vi "DrawCircle.vi"(6 "Phase":dbl step=0.1, 8 "Eccentricity":dbl min=0.0 step=0.05, 9 "No Of Points":i32, 10 "Radius":dbl, 11 "Center":cluster{"X":dbl, "Y":dbl}) -> (3 "Array":dbl[][](array[numeric]))   [LabVIEW 2017]
uses:
  <vilib>/Analysis/1siggen.llb/Ramp Pattern by Samples.vi
  <vilib>/Analysis/NI_AALBase.lvlib
panel:
  out "Array 3":i32[](array[numeric])
  out "XY Graph":cluster{"X":dbl, "Y":dbl}[](graph)
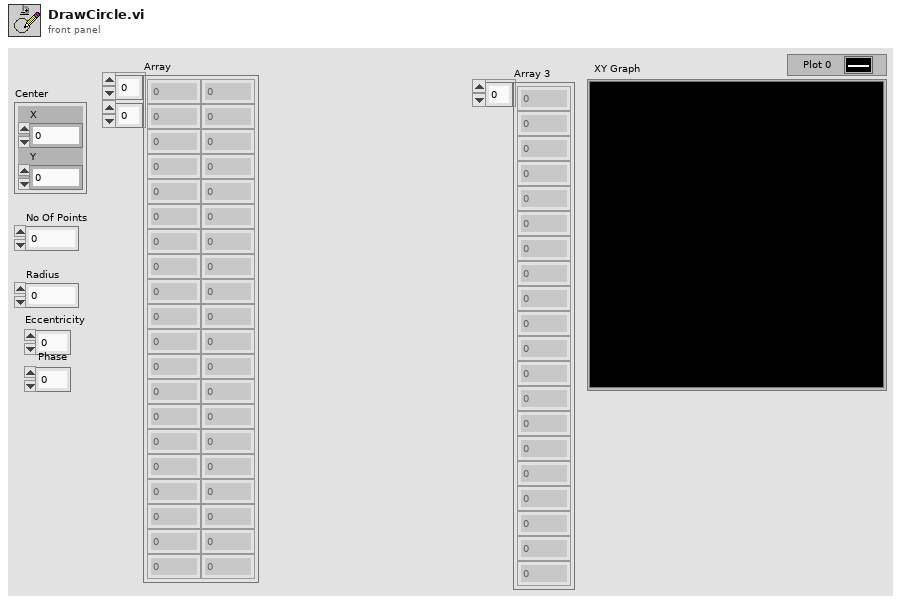
[diagram p1: front panel]
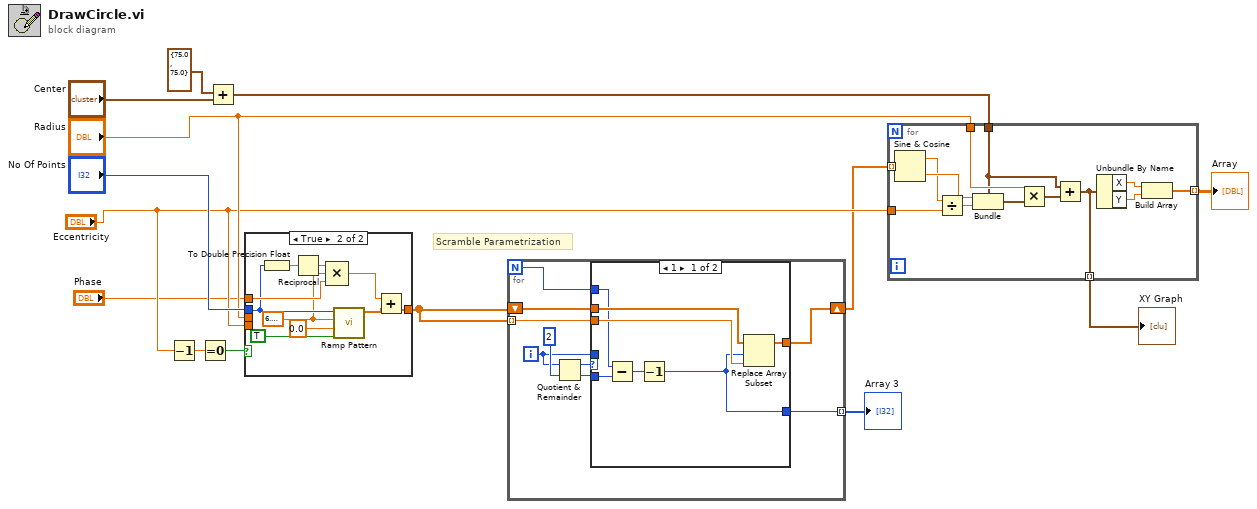
[diagram p0: block diagram]
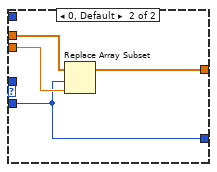
[diagram p2: hidden frame]
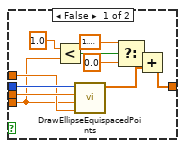
[diagram p3: hidden frame]
diagram:
  # "Scramble Parametrization"
  n1 = Decrement(x="Eccentricity") -> (x-1=w8:dbl)
  n2 = Equal To 0?(x=w8) -> (x = 0?=w10:bool)
  n3 = Add(x=cluster{"X":dbl, "Y":dbl} {"X"=75.0, "Y"=75.0} ("y"), y="Center") -> (x+y=w12:cluster{"X":dbl, "Y":dbl})
  n4 = case shown="True" w10 {
    tunnel: "No Of Points" -> [w25 w29]
    tunnel: [w18 w32] -> w2
    tunnel: "Radius" -> [w24 _]
    tunnel: "Eccentricity" -> [w15 _]
    tunnel: "Phase" -> [w23 w31]
    frame False {
      n5 = Less?(x=1.0 ("f"), y=w15) -> (x < y?=w17:bool)
      n6 = call "DrawEllipseEquispacedPoints.vi"("Phase"=w23, "Eccentricity"=w15, "Radius"=w24, "Points"=w25) -> ("Array"=w19:dbl[])  [unwired: 7 in]
      n7 = Select(t=1.5707963267948966, s=w17, f=0.0) -> (s? t:f=w20:dbl)
      n8 = Add(x=w20, y=w19) -> (x+y=w18:dbl[])
    }
    frame True {
      w26 = 6.283185307179586
      n9 = To Double Precision Float(number=w29) -> (double precision float=w27:dbl)
      n10 = Reciprocal(x=w27) -> (1/x=w28:dbl)
      n11 = Compound Arithmetic op=MULTIPLY(w28, w26, w31) -> (w30:dbl)
      n12 = call-poly <vilib>:"Ramp Pattern.vi"("exclude end?"=TRUE, "start"=0.0, "end"=w26, "samples"=w29) -> ("Ramp Pattern"=w33:dbl[])  [unwired: 6 in, 1 out]
      n13 = Add(x=w30, y=w33) -> (x+y=w32:dbl[])
    }
  }
  n14 = for {
    N -> [w38]
    tunnel: w2 -> [w40] mode=indexing
    tunnel: [w37] -> w4 mode=indexing
    shift-right: [w39] -> w1
    shift-left: w2 -> [w41]
    i -> [w42]
    n15 = Quotient & Remainder(x=w42, y=2) -> (x-y*floor(x/y)=w44:i32, floor(x/y)=w36:i32)
    n16 = case shown="1" w44 {
      tunnel: w42 -> [_ _]
      tunnel: w41 -> [w49 w55]
      tunnel: w40 -> [w51 w54]
      tunnel: [w50 w53] -> w39
      tunnel: w38 -> [w48 _]
      tunnel: [w45 w52] -> w37
      tunnel: w36 -> [w47 w52]
      frame 1 {
        n17 = Subtract(x=w48, y=w47) -> (x-y=w46:i32)
        n18 = Decrement(x=w46) -> (x-1=w45:i32)
        n19 = Replace Array Subset(array=w49, new element=w51, index=w45) -> (w50:dbl[])
      }
      frame 0, Default {
        n20 = Replace Array Subset(array=w55, new element=w54, index=w52) -> (w53:dbl[])
      }
    }
  }
  "Array 3" <- w4
  n21 = for {
    tunnel: w12 -> [w64]
    tunnel: "Radius" -> [w68]
    tunnel: [w61] -> w3 mode=indexing
    tunnel: "Eccentricity" -> [w58]
    tunnel: w1 -> [w57] mode=indexing
    tunnel: [w56] -> w5 mode=indexing
    n22 = Sine & Cosine(0:w57) -> (1:w60:dbl, 2:w67:dbl)
    n23 = Divide(x=w60, y=w58) -> (x/y=w59:dbl)
    n24 = Bundle(cluster=w64, "X"=w67, "Y"=w59) -> (w66:cluster{"X":dbl, "Y":dbl})
    n25 = Multiply(x=w68, y=w66) -> (x*y=w65:cluster{"X":dbl, "Y":dbl})
    n26 = Add(x=w64, y=w65) -> (x+y=w56:cluster{"X":dbl, "Y":dbl})
    n27 = Unbundle By Name(w56) -> ("X"=w63:dbl, "Y"=w62:dbl)
    n28 = Build Array(w63, w62) -> (w61:dbl[])
  }
  "Array" <- w3
  "XY Graph" <- w5
